vi "IMMU - Read Magnetometer Val.vi"(8 "error in (no error)":errorcluster, 11 "I2C Ref In":T1={"myRIO Reference"={"myRIO Model"=enum."Unknown", "myRIO Hardware Reference"={"Generic FPGA Reference"=refnum, "Allow multiple opens"=FALSE}}, "I2C Channels Enum"=enum."Not Connected", "I2C Configuration"={"I2C Transfer Rate"=enum."Fast mode (400 kbps)"}}) -> (0 "error out":errorcluster, 2 "Magnetometer Flux Out (uT)":dbl[](array[numeric]), 3 "I2C Ref Out":T1={"myRIO Reference"={"myRIO Model"=enum."Unknown", "myRIO Hardware Reference"={"Generic FPGA Reference"=refnum, "Allow multiple opens"=FALSE}}, "I2C Channels Enum"=enum."Not Connected", "I2C Configuration"={"I2C Transfer Rate"=enum."Fast mode (400 kbps)"}})   [LabVIEW 2021]
uses:
  <vilib>/myRIO/Instrument Drivers/Onboard IO/I2C/typedefs/I2C Reference.ctl
  <vilib>/myRIO/Common/Instrument Driver Framework/Utilities/typedefs/myRIO Generic Hardware Reference.ctl
  <vilib>/myRIO/Common/Instrument Driver Framework/Utilities/typedefs/Hardware Version Enum.ctl
  <vilib>/myRIO/Common/Instrument Driver Framework/Utilities/typedefs/myRIO v1.0 Reference.ctl
  <vilib>/myRIO/Common/Instrument Driver Framework/Utilities/typedefs/Generic FPGA Reference.ctl
  <vilib>/myRIO/Common/Instrument Driver Framework/myRIO v1.0/I2C/typedefs/I2C Channels Enum.ctl
  <vilib>/myRIO/Instrument Drivers/Onboard IO/I2C/typedefs/I2C Configuration.ctl
  <vilib>/myRIO/Instrument Drivers/Onboard IO/I2C/typedefs/I2C Transfer Rate.ctl
  <vilib>/Utility/error.llb/Error Cluster From Error Code.vi
  <vilib>/myRIO/Common/Instrument Driver Framework/myRIO v1.0/I2C/vis/myRIO v1.0 Write I2C.vi
  <vilib>/myRIO/Common/Instrument Driver Framework/myRIO v1.0/I2C/vis/myRIO v1.0 Read I2C.vi
  <vilib>/myRIO/Instrument Drivers/Onboard IO/I2C/I2C.lvlib
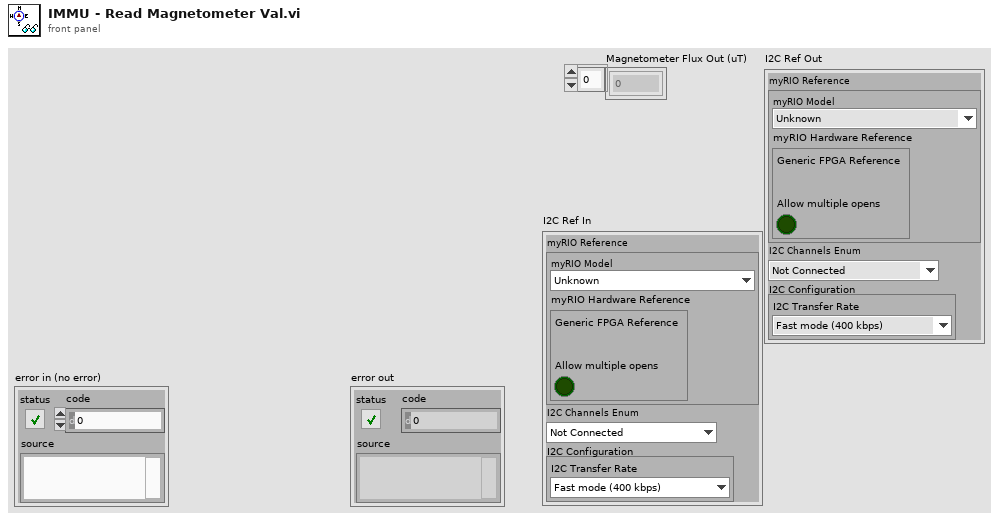
[diagram p1: front panel]
types:
  T1 = typedef "I2C.lvlib/I2C Reference.ctl" = cluster{"myRIO Reference":T2, "I2C Channels Enum":T6, "I2C Configuration":T7}
  T2 = typedef "myRIO Generic Hardware Reference.ctl" = cluster{"myRIO Model":T3, "myRIO Hardware Reference":T4}
  T3 = typedef "Hardware Version Enum.ctl" = enum16{"Unknown", "myRIO-1900", "myRIO-1950", "roboRIO", "NI ELVIS RIO CM", "ELVIS III"}
  T4 = typedef "myRIO v1.0 Reference.ctl" = cluster{"Generic FPGA Reference":T5, "Allow multiple opens":bool}
  T5 = typedef "Generic FPGA Reference.ctl" = refnum<k20>
  T6 = typedef "I2C Channels Enum.ctl" = enum16{"Not Connected", "A/I2C", "B/I2C", "I2C/I2C"}
  T7 = typedef "I2C.lvlib/I2C Configuration.ctl" = cluster{"I2C Transfer Rate":T8}
  T8 = typedef "I2C.lvlib/I2C Transfer Rate.ctl" = enum16{"Standard mode (100 kbps)", "Fast mode (400 kbps)"}
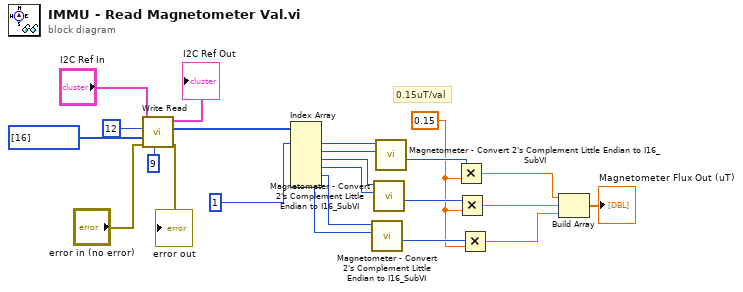
[diagram p0: block diagram]
diagram:
  w6 = 0.15
  # "0.15uT/val"
  n1 = call <vilib>:"Write Read.vi"("Byte Count"=u32 9, "error in (no error)"="error in (no error)", "Bytes to Write"=u8[] [16], "Slave Address (7-bit)"=u8 12, "I2C Ref In"="I2C Ref In") -> ("error out"=→"error out":errorcluster, "Bytes Read"=w13:u8[], "I2C Ref Out"=→"I2C Ref Out":T1)  [unwired: 3 in]
  n2 = Index Array(array=w13, index #1=1 ("index")) -> (element #1=w16:u8, element #2=w15:u8, element #3=w18:u8, element #4=w19:u8, element #5=w21:u8, element #6=w22:u8)  [unwired: 5 in]
  n3 = call "Magnetometer - Convert 2's Complement Little Endian to I16_SubVI.vi"("High Byte"=w22, "Low Byte"=w21) -> ("Output I16"=w23:i16)  [unwired: 9 in]
  n4 = call "Magnetometer - Convert 2's Complement Little Endian to I16_SubVI.vi"("High Byte"=w19, "Low Byte"=w18) -> ("Output I16"=w20:i16)  [unwired: 9 in]
  n5 = call "Magnetometer - Convert 2's Complement Little Endian to I16_SubVI.vi"("High Byte"=w15, "Low Byte"=w16) -> ("Output I16"=w17:i16)  [unwired: 9 in]
  n6 = Multiply(x=w17, y=w6) -> (x*y=w5:dbl)
  n7 = Multiply(x=w20, y=w6) -> (x*y=w4:dbl)
  n8 = Multiply(x=w23, y=w6) -> (x*y=w3:dbl)
  n9 = Build Array(w5, w4, w3) -> (→"Magnetometer Flux Out (uT)":dbl[])
